vi "PQCopyCount.vi"(6 "error in (no error)":errorcluster, 8 "optional clause":string, 9 "CountClumn":string="id", 10 "table":string, 11 "conn":u32) -> (0 "DatabaseMesssageCluster":T1, 2 "Count":i32, 3 "conn_out":u32, 4 "error out":errorcluster)   [LabVIEW 2019, in "libpqutility.lvlib"]
doc: "Count is needet to initialise\nresultset Array in CopyOut make shure\nto use PQCopyCount to get the number of Rows\nexpectet from CopyOut"
uses:
  libpqutility.lvlib
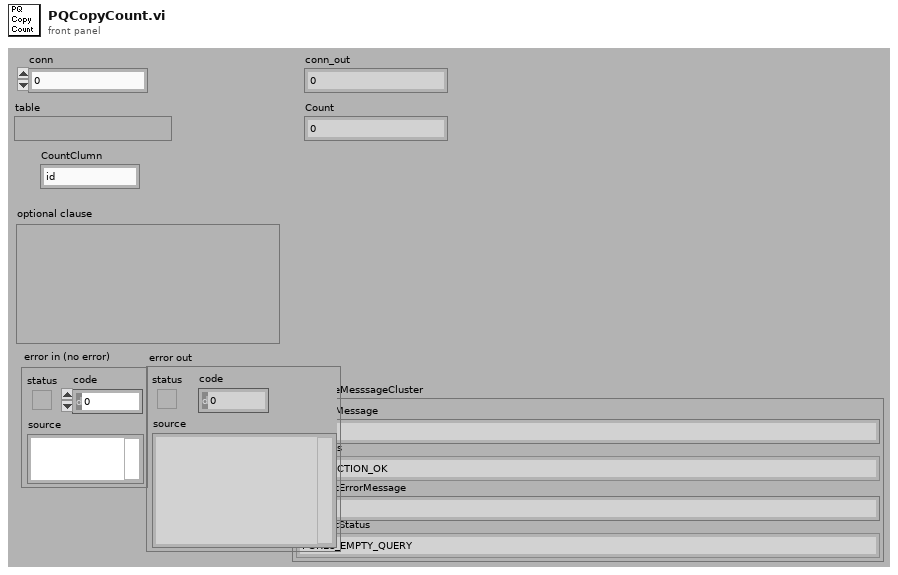
[diagram p1: front panel]
types:
  T1 = cluster{"PQerrorMessage":string, "PQStatus":enum16{"CONNECTION_OK", "CONNECTION_BAD", "CONNECTION_STARTED", "CONNECTION_MADE", "CONNECTION_AWAITING_RESPONSE", "CONNECTION_AUTH_OK", "CONNECTION_SETENV", "CONNECTION_SSL_STARTUP", "CONNECTION_NEEDED"}, "PQresultErrorMessage":string, "PQresultStatus":enum16{"PGRES_EMPTY_QUERY", "PGRES_COMMAND_OK", "PGRES_TUPLES_OK", "PGRES_COPY_OUT", "PGRES_COPY_IN", "PGRES_BAD_RESPONSE", "PGRES_NONFATAL_ERROR", "PGRES_FATAL_ERROR"}}
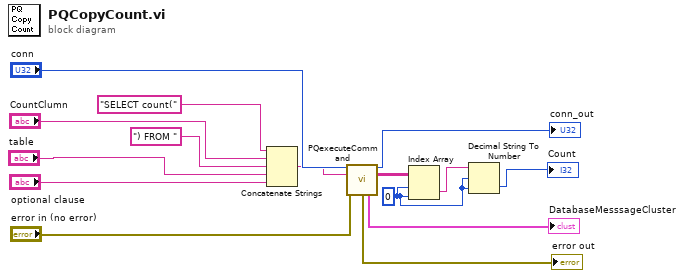
[diagram p0: block diagram]
diagram:
  w2 = 0 ("Index")
  n1 = Concatenate Strings("SELECT count(" ("String"), "CountClumn", ") FROM " ("String"), "table", "optional clause") -> (w4:string)
  n2 = call "PQexecuteCommand.vi"("conn"="conn", "Command"=w4, "error in (no error)"="error in (no error)") -> ("conn_out"=→"conn_out":u32, "Data"=w6:string[][], "error out"=→"error out":errorcluster, "DatabaseMesssageCluster"=→"DatabaseMesssageCluster":T1)  [unwired: 6 in, 3 out]
  n3 = Index Array(array=w6, index (row)=w2, index (col)=w2) -> (element=w5:string)
  n4 = Decimal String To Number(string=w5, offset=w2, default (0L)=w2) -> (number=→"Count":i32)  [unwired: 1 out]
